vi "shuffleBlockCondition (SubVI).vi"(3 "randomize?(no:F)":bool, 5 "Protocol in":T1) -> (2 "Protocol out":T1)   [LabVIEW 2021]
uses:
  ctlProtocol.ctl
  ctlProtocolSubID.ctl
  ctlBlockOrder.ctl
  ctrBlockCondition.ctl
  <vilib>/Analysis/1siggen.llb/Riffle Array (I32) (obs 2012).vi
  <vilib>/Analysis/NI_AALBase.lvlib
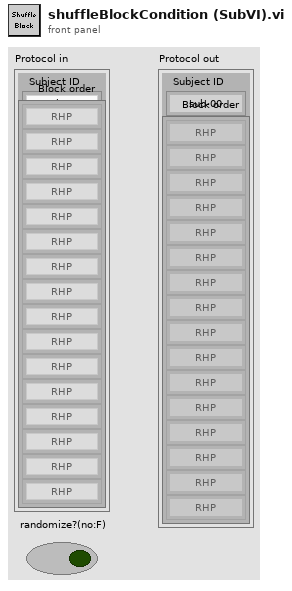
[diagram p1: front panel]
types:
  T1 = typedef "ctlProtocol.ctl" = cluster{"Subject ID":T2, "Block order":T3}
  T2 = typedef "ctlProtocolSubID.ctl" = enum16{"sub-00", "sub-01", "sub-02", "sub-03", "sub-04", "sub-05", "sub-06", "sub-07", "sub-08", "sub-09", "sub-10", "sub-11", "sub-12", "sub-13", "sub-14", "sub-15", "sub-16", "sub-17", "sub-18", "sub-19", "sub-20", "sub-21", "sub-22", "sub-23", "sub-24", "sub-25", "sub-26", "sub-27", "sub-28", "sub-29", "sub-30", "sub-31", "sub-32", "sub-33", "sub-34", "sub-35", "sub-36", "sub-37", "sub-38", "sub-39", "sub-40"}
  T3 = typedef "ctlBlockOrder.ctl" = T4[]
  T4 = typedef "ctrBlockCondition.ctl" = enum16{"famDrop", "preDrop", "famTask", "RHP", "RLD", "RHD", "LHP", "LLD", "LHD", "UR", "UL", "pstDrop"}
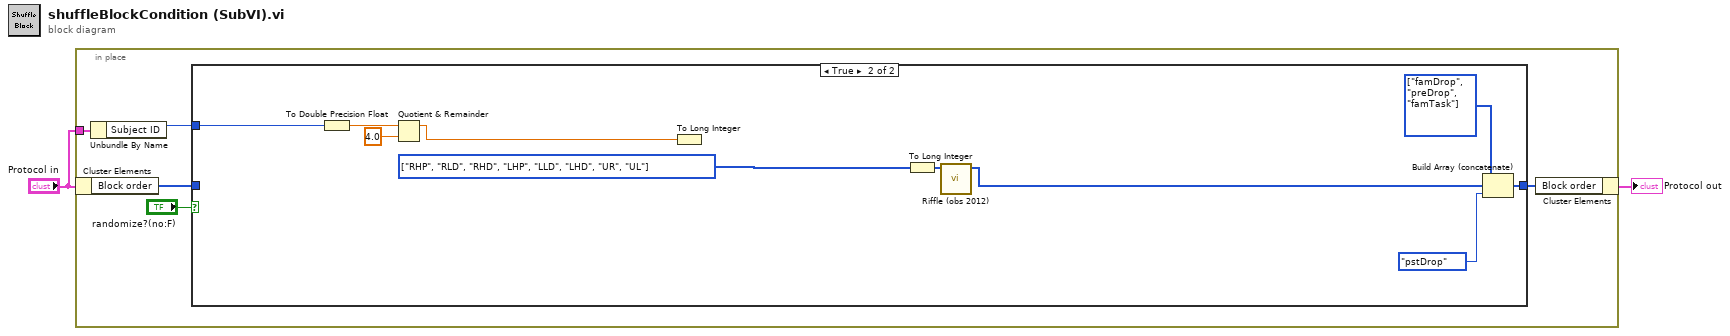
[diagram p0: block diagram]
diagram:
  n1 = in-place {
    in-place-border: "Protocol in" -> [w5]
    n2 = in-place-cluster #1("Protocol in") -> ("Block order"=w7:T3)
    n3 = Unbundle By Name(w5) -> ("Subject ID"=w4:T2)
    n4 = case shown="True" "randomize?(no:F)" {
      tunnel: w7 -> [w8 _]
      tunnel: [w8 w18] -> w3
      tunnel: w4 -> [_ w17]
      frame False {
      }
      frame True {
        w13 = T4[] [enum."RHP", enum."RLD", enum."RHD", enum."LHP", enum."LLD", enum."LHD", enum."UR", enum."UL"] items=["famDrop", "preDrop", "famTask", "RHP", "RLD", "RHD", "LHP", "LLD", "LHD", "UR", "UL", "pstDrop"]
        w16 = T3 [enum."famDrop", enum."preDrop", enum."famTask"] items=["famDrop", "preDrop", "famTask", "RHP", "RLD", "RHD", "LHP", "LLD", "LHD", "UR", "UL", "pstDrop"] ("Block order")
        n5 = To Double Precision Float(number=w17) -> (double precision float=w12:dbl)
        n6 = Quotient & Remainder(x=w12, y=4.0) -> (x-y*floor(x/y)=w10:dbl)  [unwired: 1 out]
        n7 = To Long Integer(number=w10) -> ()  [unwired: 1 out]
        n8 = To Long Integer(number=w13) -> (32bit integer=w14:i32[])
        n9 = call-poly <vilib>:"Riffle (obs 2012).vi"("X"=w14) -> ("Riffled {X}"=w9:i32[])  [unwired: 8 in, 2 out]
        n10 = Build Array (concatenate)(w16, w9, ctrBlockCondition."pstDrop" ("Block Condition")) -> (w18:i32[])
      }
    }
    n11 = in-place-cluster #1("Block order"=w3) -> (→"Protocol out":T1)
  }
